vi "Get Object Parameter - Numeric.vi"(8 "error in (no error)":errorcluster, 9 "Default Value if JSON Null":dbl, 10 "Parameter Name":string, 11 "JSON Tree In (JSON Object)":variant) -> (0 "error out":errorcluster, 1 "is JSON Null?":bool, 2 "Double Value":dbl, 3 "JSON Tree Out Passthrough":variant)   [LabVIEW 2013, in "i3-json.lvlib"]
doc: "Get a named parameter from a JSON Tree Object"
uses:
  i3-json.lvlib
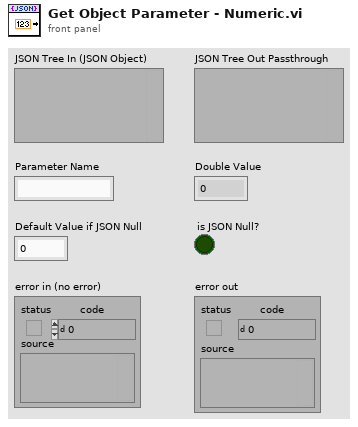
[diagram p1: front panel]
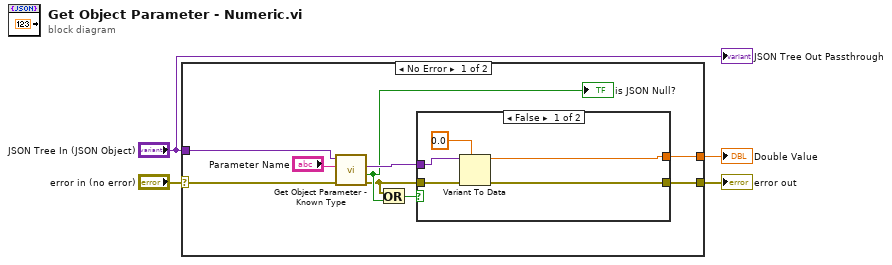
[diagram p0: block diagram]
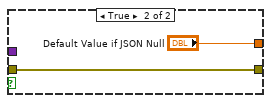
[diagram p2: hidden frame]
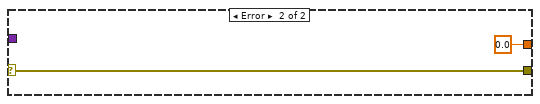
[diagram p3: hidden frame]
diagram:
  n1 = case shown="No Error" "error in (no error)" {
    selector: "error in (no error)" -> [w12 w22]
    tunnel: [w10 w22] -> w3
    tunnel: "JSON Tree In (JSON Object)" -> [w13 _]
    tunnel: [w7 0.0 ("Default Value if JSON Null")] -> w2
    frame No Error {
      n2 = call "Get Object Parameter - Known Type.vi"("error in (no error)"=w12, "Parameter Name"="Parameter Name", "JSON Tree In (JSON Object)"=w13) -> ("error out"=w5:errorcluster, "is JSON Null?"=w8:bool, "Value"=w9:variant)  [unwired: 3 in, 3 out]
      "is JSON Null?" <- w8
      n3 = Or(x=w5, y=w8) -> (x .or. y?=w11:bool)
      n4 = case shown="False" w11 {
        tunnel: w5 -> [w18 w20]
        tunnel: [w15 w20] -> w10
        tunnel: w9 -> [w17 _]
        tunnel: [w16 "Default Value if JSON Null"] -> w7
        frame False {
          n5 = Variant To Data(error in=w18, type=0.0 ("Double Value"), Variant=w17) -> (data=w16:dbl, error out=w15:errorcluster)
        }
        frame True {
        }
      }
    }
    frame Error {
    }
  }
  "error out" <- w3
  "Double Value" <- w2
  "JSON Tree Out Passthrough" <- "JSON Tree In (JSON Object)"
